vi "Demo Main.vi"() -> ()   [LabVIEW 2020, in "VolatusDemo.lvlib"]
uses:
  VolatusDemo.lvlib
  Volatus/Event.ctl
  Volatus/Event Level.ctl
  DemoApp/DemoApp.lvclass
  C:/dev/lv20CE/relink/lv-volatus/Volatus/App/App.lvclass
  Volatus/Volatus.lvlib
panel:
  out "Events":T1[](array[typedef]) {"Time Stamp" format="%<%.3X %x>T"}
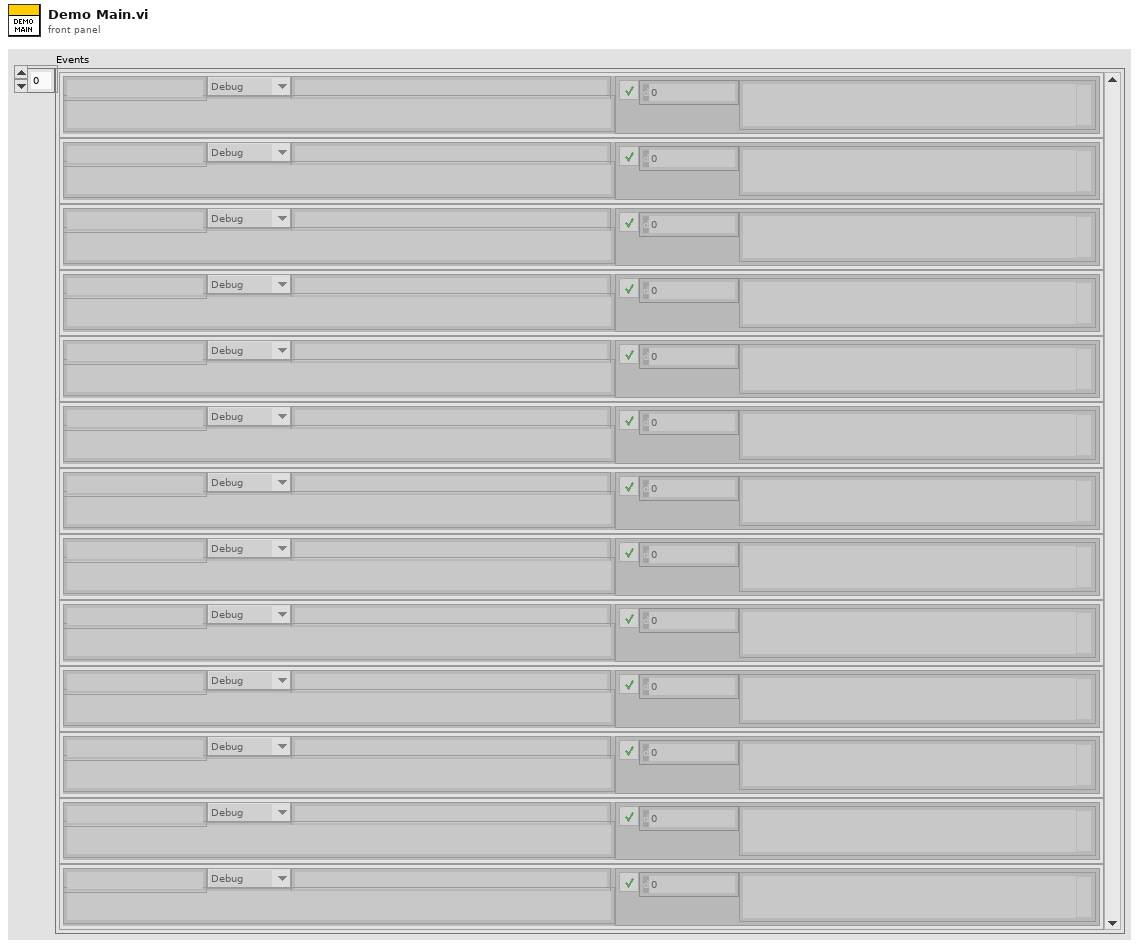
[diagram p1: front panel]
types:
  T1 = typedef "Volatus.lvlib/Event.ctl" = cluster{"Level":T2, "Context":string, "Message":string, "Error":errorcluster, "Time Stamp":timestamp}
  T2 = typedef "Volatus.lvlib/Event Level.ctl" = enum16{"Debug", "Info", "Warning", "Error"}
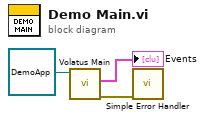
[diagram p0: block diagram]
diagram:
  n1 = call "Volatus Main.vi"("App in"=refnum<class "DemoApp.lvclass"> refnum ("VolatusDemo.lvlib:DemoApp.lvclass")) -> ("error out"=w2:errorcluster, "Events"=→"Events":T1[])  [unwired: 9 in]
  n2 = call <vilib>:"Simple Error Handler.vi"("error in (no error)"=w2) -> ()  [unwired: 4 in, 5 out]
